vi "按钮与开关.vi"() -> ()   [LabVIEW 2013]
panel:
  in  "确定按钮":bool
  in  "停止按钮":bool
  out "开关指示灯":bool
  out "按钮指示灯":bool
  in  "翘板开关":bool
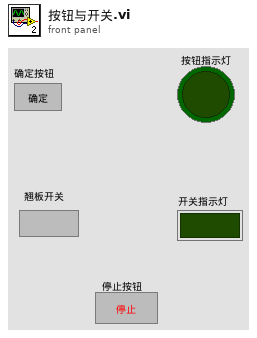
[diagram p1: front panel]
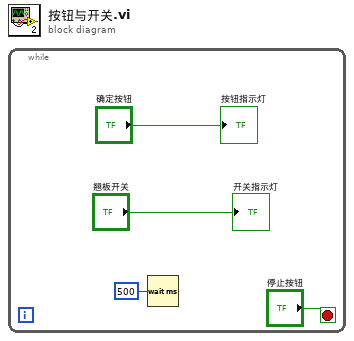
[diagram p0: block diagram]
diagram:
  n1 = while {
    stop <- "停止按钮" stop-if-true
    n2 = Wait (ms)(milliseconds to wait=u32 500 ("等待时间（毫秒）")) -> ()  [unwired: 1 out]
    "按钮指示灯" <- "确定按钮"
    "开关指示灯" <- "翘板开关"
  }
